vi "example_cmd.vi"() -> ()   [LabVIEW 2013]
doc: "This examples launches the cmd.exe process and allows you to send strings via stdin, while asynchronously listening to stdout and stderr \n\nCalling \"exit\" in CmdIn will stop the cmd.exe instance and stop this VI. You can leverage this by adding a final exit line after the command(s)\nyou wish to send to have this VI auto-terminate upon completion."
uses:
  dotnet_system_exec/dotnet_system_exec.lvclass
panel:
  in  "working directory":path=path "c:/"
  out "StdErr":string
  out "StdOut":string
  in  "Send":bool
  in  "Cmd In (can include multiple lines)":string="dir"
  in  "Stop":bool
  # "This examples launches the cmd.exe process and allows you to send strings via stdin, while asynchronously listening to stdout and stderr  \n\nCalling \"exit\" in CmdIn will stop the cmd.exe instance and stop this VI. You can leverage this by adding a final exit line after the command(s)\nyou wish to send to have this VI auto-terminate upon completion."
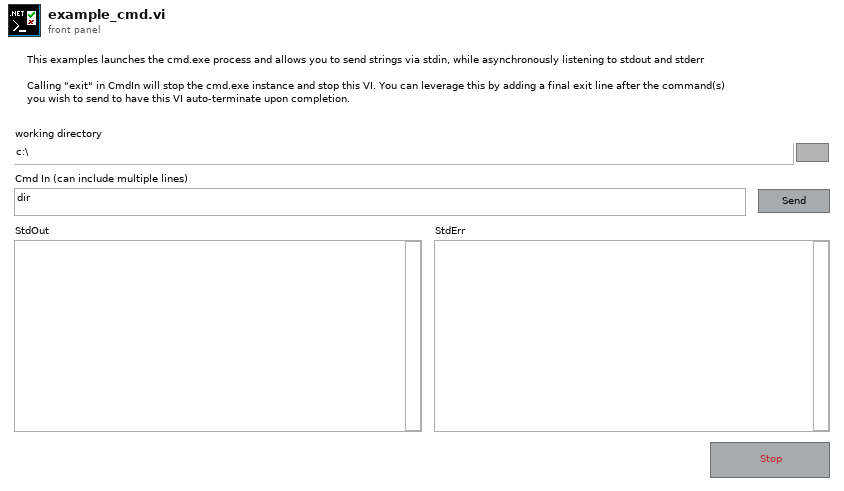
[diagram p1: front panel]
types:
  T1 = cluster{"stdout event":refnum<user-event>, "stderr event":refnum<user-event>, "process_exit event":refnum<user-event>}
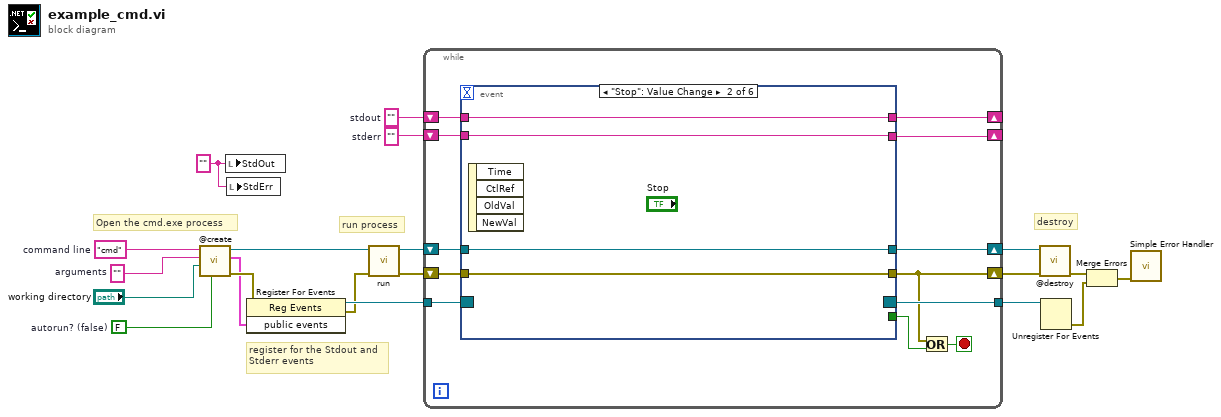
[diagram p0: block diagram]
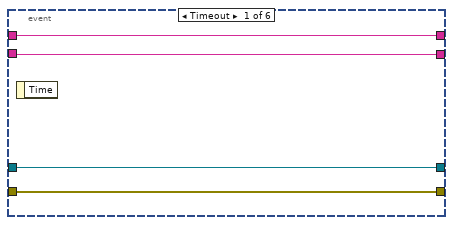
[diagram p2: hidden frame]
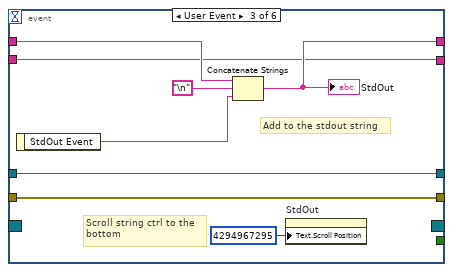
[diagram p3: hidden frame]
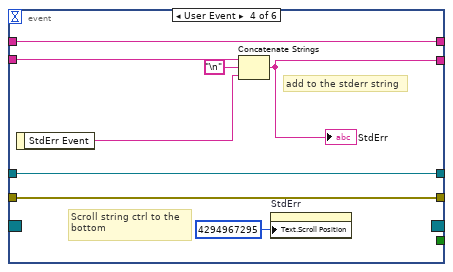
[diagram p4: hidden frame]
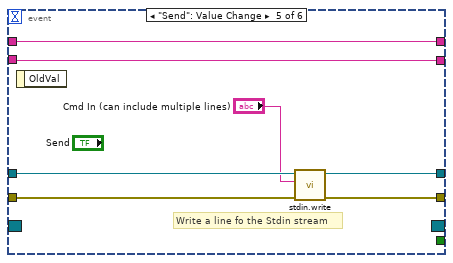
[diagram p5: hidden frame]
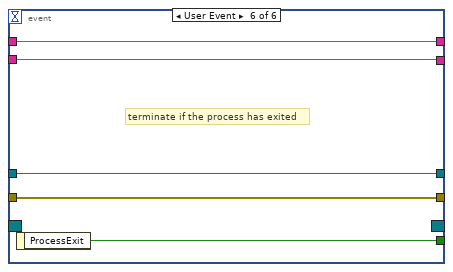
[diagram p6: hidden frame]
diagram:
  w1 = FALSE  # autorun? (false)
  w2 = "" ("Process File Name")
  w4 = ""  # stderr
  w9 = ""  # arguments
  w10 = ""  # stdout
  w11 = "cmd"  # command line
  # "destroy"
  # "register for the Stdout and\nStderr events"
  # "run process"
  # "Open the cmd.exe process"
  n1 = call "@create.vi"("autorun? (false)"=w1, "working directory (c:\\)"="working directory", "arguments (\"\")"=w9, "command line (cmd.exe)"=w11) -> ("error out"=w7:errorcluster, "public events"=w5:T1, "dotnet_system_exec out"=w18:refnum<class "dotnet_system_exec.lvclass">)  [unwired: 5 in]
  n2 = local write "StdOut"(w2) -> ()
  n3 = local write "StdErr"(w2) -> ()
  n4 = register-events(error in=w7, w5) -> (reference out=w17:refnum<event-registration>, error out=w6:errorcluster)  [unwired: 1 in]
  n5 = call "run.vi"("error in (no error)"=w6, "dotnet_system_exec in"=w18) -> ("error out"=w8:errorcluster, "dotnet_system_exec out"=w20:refnum<class "dotnet_system_exec.lvclass">)  [unwired: 8 in]
  n6 = while {
    shift-right: [w32] -> w19
    shift-left: w20 -> [w31]
    shift-right: [w22] -> w15
    shift-left: w8 -> [w30]
    tunnel: w17 -> [w29]
    tunnel: [w28] -> w16
    shift-right: [w26] -> _
    shift-left: w10 -> [w27]
    shift-right: [w24] -> _
    shift-left: w4 -> [w25]
    stop <- w21 stop-if-true
    n7 = event shown="[1] \"Stop\": Value Change" {
      selector: w29 -> [_ _ _ _ _ _]
      dyn-events: [_ _ _ _ _ _] -> w28
      timeout: _ -> [_ _ _ _ _ _]
      tunnel: [w36 w41 w49 w57 w64 w66] -> w32
      tunnel: w31 -> [w36 w41 w49 w57 w63 w66]
      tunnel: w30 -> [w35 w40 w48 w56 w61 w65]
      tunnel: [w35 w40 w48 w56 w62 w65] -> w22
      tunnel: w27 -> [w34 w38 w45 w52 w59 w67]
      tunnel: [w34 w38 w46 w52 w59 w67] -> w26
      tunnel: [_ TRUE _ _ _ w69] -> w23
      tunnel: w25 -> [w33 w37 w43 w53 w58 w68]
      tunnel: [w33 w37 w43 w51 w58 w68] -> w24
      event Timeout {
        n8 = event-data() -> ()  [unwired: 1 in, 1 out]
      }
      event "Stop": Value Change {
        n9 = event-data() -> ()  [unwired: 1 in, 4 out]
      }
      event User Event {
        # "Scroll string ctrl to the \nbottom"
        # "Add to the stdout string"
        n10 = event-data() -> ("StdOut Event"=w44:string)  [unwired: 1 in]
        n11 = Concatenate Strings(w45, "\n", w44) -> (w46:string)
        "StdOut" <- w46
        n12 = property on="StdOut" class="Str"("Text.Scroll Position"=u32 4294967295) -> ()  [unwired: 2 in, 2 out]
      }
      event User Event {
        # "Scroll string ctrl to the \nbottom"
        # "add to the stderr string"
        n13 = event-data() -> ("StdErr Event"=w54:string)  [unwired: 1 in]
        n14 = Concatenate Strings(w53, "\n", w54) -> (w51:string)
        "StdErr" <- w51
        n15 = property on="StdErr" class="Str"("Text.Scroll Position"=u32 4294967295) -> ()  [unwired: 2 in, 2 out]
      }
      event "Send": Value Change {
        # "Write a line fo the Stdin stream"
        n16 = event-data() -> ()  [unwired: 1 in, 1 out]
        n17 = call-dynamic "stdin.write.vi"("error in (no error)"=w61, "stdin"="Cmd In (can include multiple lines)", "dotnet_system_exec in"=w63) -> ("error out"=w62:errorcluster, "dotnet_system_exec out"=w64:refnum<class "dotnet_system_exec.lvclass">)  [unwired: 7 in]
      }
      event User Event {
        # "terminate if the process has exited"
        n18 = event-data() -> ("ProcessExit"=w69:bool)  [unwired: 1 in]
      }
    }
    n19 = Or(x=w22, y=w23) -> (x .or. y?=w21:bool)
  }
  n20 = call-dynamic "@destroy.vi"("error in (no error)"=w15, "dotnet_system_exec in"=w19) -> ("error out"=w14:errorcluster)  [unwired: 8 in, 1 out]
  n21 = Unregister For Events(event registration refnum=w16) -> (error out=w13:errorcluster)  [unwired: 1 in]
  n22 = Merge Errors(w14, w13) -> (w12:errorcluster)
  n23 = call <vilib>:"Simple Error Handler.vi"("error in (no error)"=w12) -> ()  [unwired: 4 in, 5 out]
